vi "PC1.vi"() -> ()   [LabVIEW 2016]
panel:
  out "String 2":string
  in  "String":string
  in  "Stop Button":bool
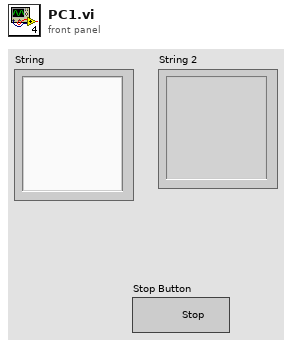
[diagram p1: front panel]
types:
  T1 = enum16{"Read", "Write", "ReadWrite", "BufferedRead", "BufferedReadWrite"}
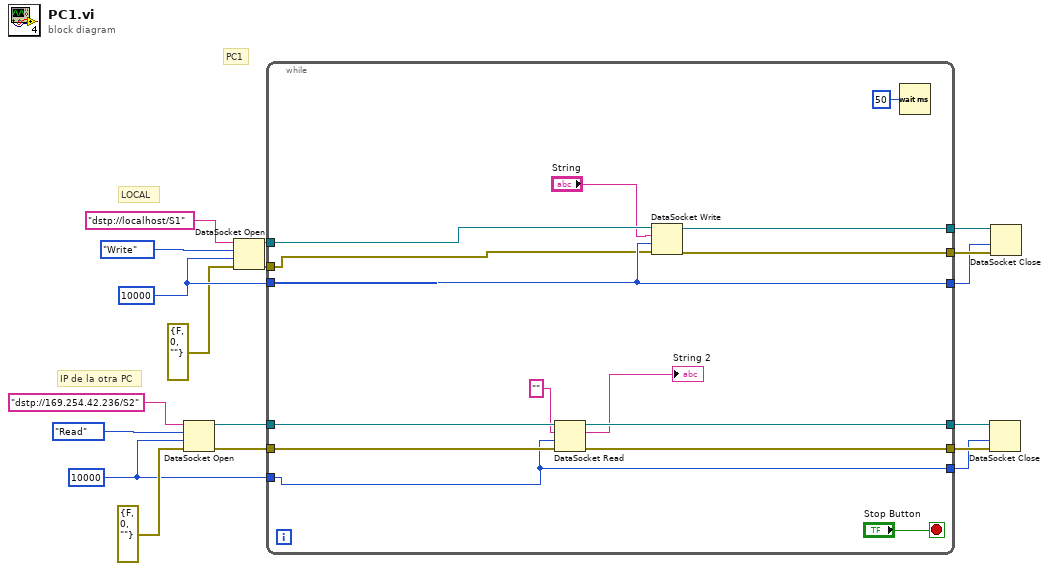
[diagram p0: block diagram]
diagram:
  w6 = 10000 ("ms timeout (10000)")
  w16 = 10000 ("ms timeout (10000)")
  # "IP de la otra PC"
  # "LOCAL"
  # "PC1"
  n1 = DataSocket Open(8:errorcluster {"status"=FALSE, "code"=0, "source"=""} ("error in (no error)"), 9:w6, 10:T1."Read" ("mode"), 11:"dstp://169.254.42.236/S2" ("URL")) -> (0:w4:errorcluster, 3:w5:refnum<k13>)
  n2 = DataSocket Open(8:errorcluster {"status"=FALSE, "code"=0, "source"=""} ("error in (no error)"), 9:w16, 10:T1."Write" ("mode"), 11:"dstp://localhost/S1" ("URL")) -> (0:w14:errorcluster, 3:w13:refnum<k13>)
  n3 = while {
    tunnel: w16 -> [w28]
    tunnel: w14 -> [w19]
    tunnel: w13 -> [w32]
    tunnel: [w30] -> w12
    tunnel: [w29] -> w11
    tunnel: [w28] -> w10
    tunnel: w6 -> [w20]
    tunnel: w5 -> [w26]
    tunnel: w4 -> [w25]
    tunnel: [w24] -> w3
    tunnel: [w23] -> w2
    tunnel: [w20] -> w1
    stop <- "Stop Button" stop-if-true
    n4 = DataSocket Read(8:w25, 9:w20, 10:"", 11:w26) -> (0:w23:errorcluster, 2:→"String 2":string, 3:w24:refnum<k13>)  [unwired: 1 in, 4 out]
    n5 = DataSocket Write(8:w19, 9:w28, 10:"String", 11:w32) -> (0:w29:errorcluster, 3:w30:refnum<k13>)  [unwired: 1 out]
    n6 = Wait (ms)(milliseconds to wait=u32 50) -> ()  [unwired: 1 out]
  }
  n7 = DataSocket Close(8:w2, 9:w1, 11:w3) -> ()  [unwired: 2 out]
  n8 = DataSocket Close(8:w11, 9:w10, 11:w12) -> ()  [unwired: 2 out]
